vi "CAL-Save Data V2.vi"(0 "Mag":dbl[](array[numeric]), 1 "Smooth Params":T1={"Method"=enum."Moving average", "MA"={"Iterations"=100, "Length"=3}, "Loess"={"Length"=21, "Type"=enum."Quadratic", "Robust"=TRUE}} {"Loess"."Length" min=1 step=1; "MA"."Length" min=1 step=1; "MA"."Iterations" min=1 step=1}, 2 "Cal Stimulus":T2={"Min Freq (Hz)"=50.0, "Max Freq (Hz)"=50000.0, "Freq Step (Hz)"=50.0, "Waveform"=enum."Chirp", "Attenuation (dB)"=20.0, "Sample Rate (Hz)"=100000.0}, 5 "Phase":dbl[](array[numeric]), 7 "Frequency":dbl[](array[numeric]), 9 "Unsmoothed Mag":dbl[](array[numeric]), 11 "error in (no error)":errorcluster, 12 "path":path, 13 "Probe Tube File":path) -> (6 "new file path":path, 15 "error out":errorcluster)   [LabVIEW 2020]
uses:
  Type Defs/Cal Stimulus.ctl
  Type Defs/Cal-Smoothing Parameters.ctl
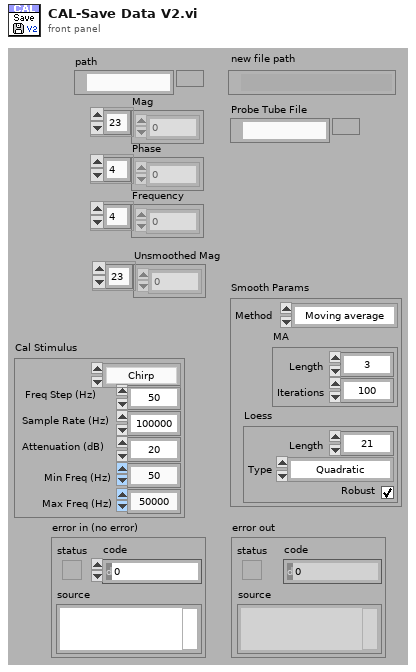
[diagram p1: front panel]
types:
  T1 = typedef "Cal-Smoothing Parameters.ctl" = cluster{"Method":enum16{"None", "Moving average", "Loess"}, "MA":cluster{"Iterations":i32, "Length":i32}, "Loess":cluster{"Length":i32, "Type":enum16{"Linear", "Quadratic"}, "Robust":bool}}
  T2 = typedef "Cal Stimulus.ctl" = cluster{"Min Freq (Hz)":dbl, "Max Freq (Hz)":dbl, "Freq Step (Hz)":dbl, "Waveform":enum16{"Chirp", "Weighted"}, "Attenuation (dB)":dbl, "Sample Rate (Hz)":dbl}
  T3 = enum16{"open", "replace", "create", "open or create", "replace or create", "replace or create with confirmation"}
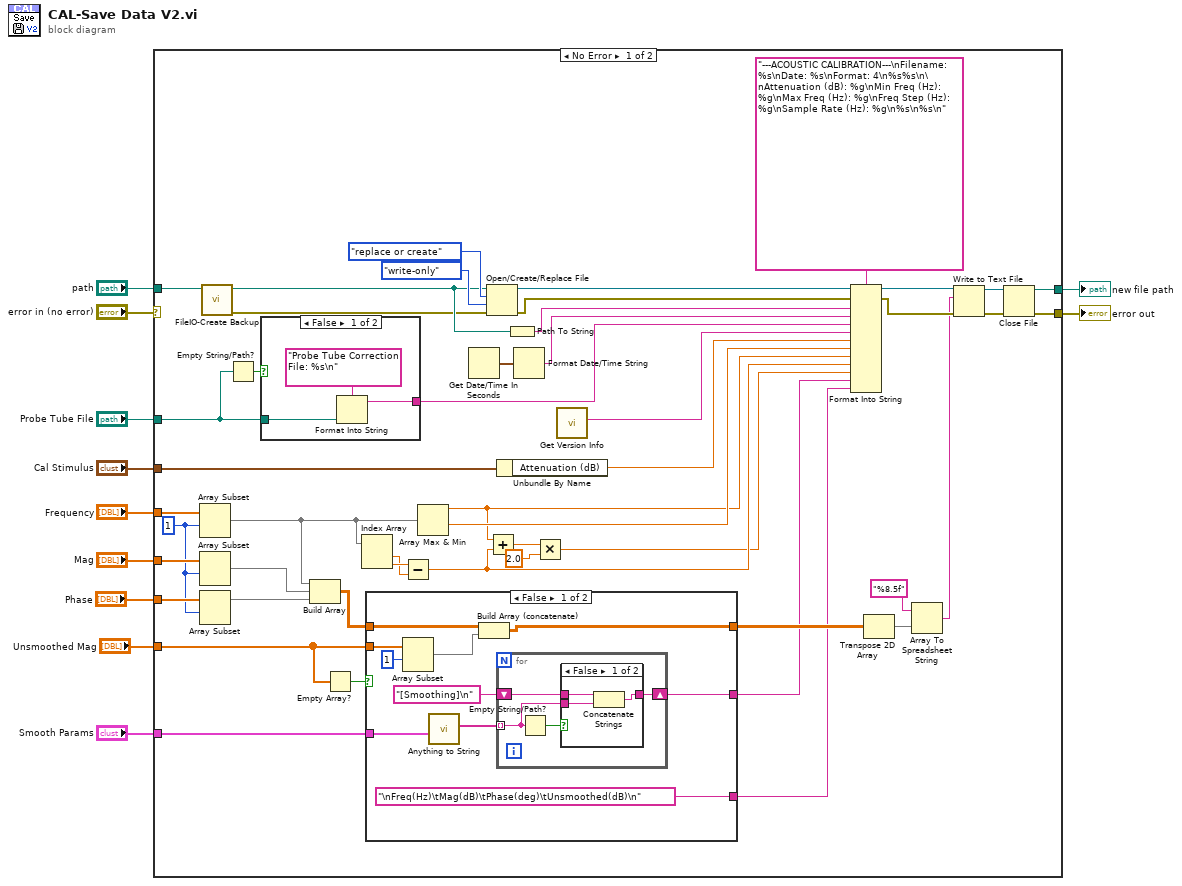
[diagram p0: block diagram]
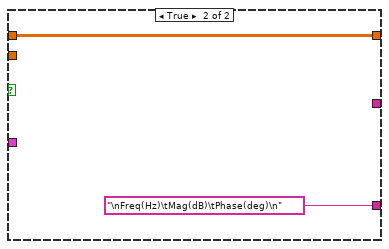
[diagram p3: hidden frame]
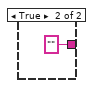
[diagram p4: hidden frame]
diagram:
  n1 = case shown="No Error" "error in (no error)" {
    selector: "error in (no error)" -> [_ w84]
    tunnel: "Phase" -> [w59 _]
    tunnel: "Mag" -> [w58 _]
    tunnel: "Frequency" -> [w39 _]
    tunnel: [w45 w84] -> w8
    tunnel: "Cal Stimulus" -> [w56 _]
    tunnel: [w44 _] -> w5
    tunnel: "path" -> [w21 _]
    tunnel: "Probe Tube File" -> [w37 _]
    tunnel: "Unsmoothed Mag" -> [w17 _]
    tunnel: "Smooth Params" -> [w14 _]
    frame No Error {
      w34 = 1 ("index")
      n2 = Array Subset(array=w39, index=w34) -> (w32:dbl[])  [unwired: 1 in]
      n3 = Array Subset(array=w58, index=w34) -> (w36:dbl[])  [unwired: 1 in]
      n4 = Array Subset(array=w59, index=w34) -> (w35:dbl[])  [unwired: 1 in]
      n5 = call "FileIO-Create Backup.vi"("Path"=w21) -> ("error out"=w19:errorcluster, "Path (thru)"=w20:path)  [unwired: 7 in, 2 out]
      n6 = Empty String/Path?(string/path=w37) -> (empty?=w38:bool)
      n7 = case shown="False" w38 {
        tunnel: w37 -> [w81 _]
        tunnel: [w80 ""] -> w24
        frame False {
          n8 = Format Into String(format string="Probe Tube Correction File: %s\n", w81) -> (resulting string=w80:string)  [unwired: 2 in, 1 out]
        }
        frame True {
        }
      }
      n9 = Build Array(w32, w36, w35) -> (w16:dbl[][])
      n10 = Empty Array?(array=w17) -> (empty?=w18:bool)
      n11 = Index Array(array=w32) -> (element #1=w30:dbl, element #2=w31:dbl)  [unwired: 2 in]
      n12 = case shown="False" w18 {
        tunnel: w17 -> [w69 _]
        tunnel: w16 -> [w67 w79]
        tunnel: [w65 w79] -> w15
        tunnel: w14 -> [w62 _]
        tunnel: [w61 _] -> w13
        tunnel: ["\nFreq(Hz)\tMag(dB)\tPhase(deg)\tUnsmoothed(dB)\n" ("format string") "\nFreq(Hz)\tMag(dB)\tPhase(deg)\n" ("format string")] -> w12
        frame False {
          n13 = Array Subset(array=w69, index=1) -> (w66:dbl[])  [unwired: 1 in]
          n14 = call "Anything to String.vi"("Anything"=w62) -> ("Strings[]"=w63:string[])  [unwired: 8 in, 2 out]
          n15 = Build Array (concatenate)(w67, w66) -> (w65:dbl[][])
          n16 = for {
            tunnel: w63 -> [w71] mode=indexing
            shift-right: [w72] -> w61
            shift-left: "[Smoothing]\n" -> [w73]
            n17 = Empty String/Path?(string/path=w71) -> (empty?=w70:bool)
            n18 = case shown="False" w70 {
              tunnel: w73 -> [w76 w77]
              tunnel: w71 -> [w75 _]
              tunnel: [w74 w77] -> w72
              frame False {
                n19 = Concatenate Strings(w76, w75) -> (w74:string)
              }
              frame True {
              }
            }
          }
        }
        frame True {
        }
      }
      n20 = Subtract(x=w31, y=w30) -> (x-y=w28:dbl)
      n21 = Array Max & Min(array=w32) -> (max value=w29:dbl, min value=w33:dbl)  [unwired: 2 out]
      n22 = Get Date/Time In Seconds() -> (seconds since 1Jan1904=w54:timestamp)
      n23 = Open/Create/Replace File(file path (use dialog)=w20, error in=w19, operation (0:open)=T3."replace or create", access (0:read/write)=enum16{"read/write", "read-only", "write-only"}."write-only") -> (refnum out=w43:refnum<file>, error out=w40:errorcluster)  [unwired: 2 in, 1 out]
      n24 = Add(x=w29, y=w28) -> (x+y=w27:dbl)
      n25 = Unbundle By Name(w56) -> ("Attenuation (dB)"=w22:dbl)
      n26 = Path To String(path=w20) -> (string=w55:string)
      n27 = Format Date/Time String(seconds (now)=w54) -> (date/time string=w53:string)  [unwired: 2 in]
      n28 = Multiply(x=w27, y=2.0) -> (x*y=w25:dbl)
      n29 = call "Get Version Info.vi"() -> ("Version Info"=w23:string)  [unwired: 10 in, 1 out]
      n30 = Format Into String(format string="---ACOUSTIC CALIBRATION---\nFilename: %s\nDate: %s\nFormat: 4\n%s%s\n\nAttenuation (dB): %g\nMin Freq (Hz): %g\nMax Freq (Hz): %g\nFreq Step (Hz): %g\nSample Rate (Hz): %g\n%s\n%s\n", initial string=w43, error in=w40, w55, w53, w24, w23, w22, w33, w29, w28, w25, w13, w12) -> (resulting string=w50:refnum<file>, error out=w49:errorcluster)
      n31 = Transpose 2D Array(2D array=w15) -> (transposed array=w51:dbl[][])
      n32 = Array To Spreadsheet String(array=w51, 3:"%8.5f" ("format (%.3f)")) -> (spreadsheet string=w48:string)  [unwired: 1 in]
      n33 = Write to Text File(file (use dialog)=w50, text=w48, error in=w49) -> (refnum out=w46:refnum<file>, error out=w47:errorcluster)  [unwired: 1 in, 1 out]
      n34 = Close File(refnum=w46, error in=w47) -> (path=w44:path, error out=w45:errorcluster)
    }
    frame Error {
    }
  }
  "error out" <- w8
  "new file path" <- w5
